vi "Test Filter Parametrized Test Cases.vi"(11 "Test Case In":refnum<class "Parameterized Test Case Test.lvclass">) -> (0 "error out":errorcluster, 3 "Test Case Out":refnum<class "Parameterized Test Case Test.lvclass">)   [LabVIEW 2020, in "Parameterized Test Case Test.lvclass"]
uses:
  Parameterized Test Case Test.lvclass
  C:/Program Files (x86)/National Instruments/LabVIEW 2020/vi.lib/Astemes/LUnit/Test Case.lvclass
  <vilib>/Astemes/LUnit/Test Case.lvclass/Test Case.ctl
  399136ac-e113-4bca-be3a-8dde4e32c814.vi
  <vilib>/Astemes/LUnit/Palette/Pass If.vi
  <vilib>/Astemes/LUnit/Append Fail Result.vi
  <vilib>/Astemes/LUnit/Append Pass Result.vi
  <vilib>/Astemes/LUnit/Run In UI.vi
  <vilib>/Utility/error.llb/Clear Errors.vi
  source/Parameterized Test Case/Parameterized Test Case.lvclass
  <vilib>/Astemes/LUnit/Test Suite.lvclass
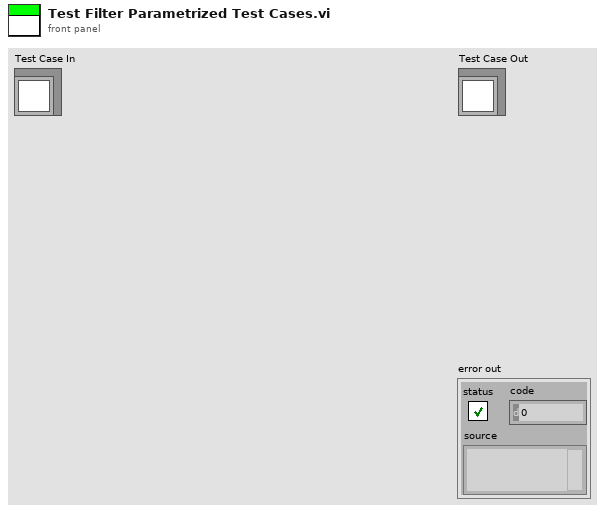
[diagram p1: front panel]
types:
  T1 = cluster{"Name":string, "Message":string, "Description":string, "Status":enum16{"", "Passed", "Failed", "Error", "Skipped", "Setup Error", "Broken", "Teardown Error"}, "Result Type":enum16{"Test Case", "Test Suite", "Test Run", "Pass", "Fail", "Skip", "Pass if", "Fail if", "Pass if Error", "Fail if Error", "Pass if Equal", "Fail if Equal"}, "Execution Time":dbl}[]
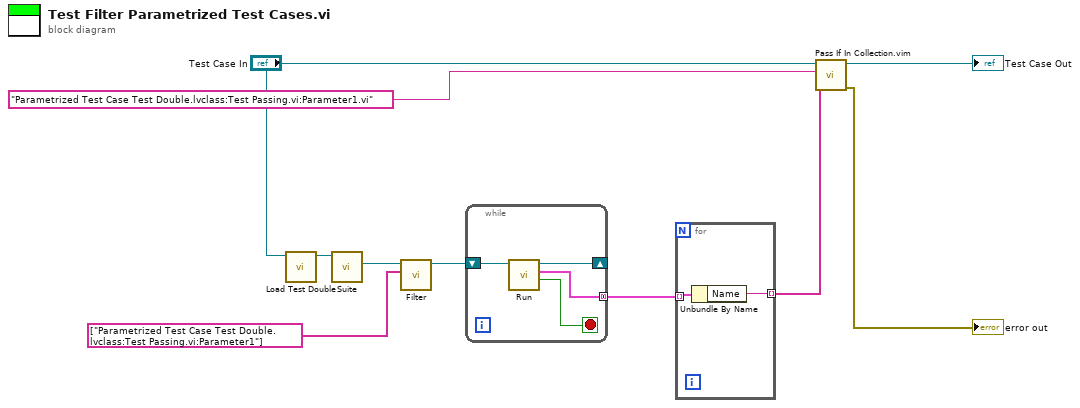
[diagram p0: block diagram]
diagram:
  n1 = call "Load Test Double.vi"("Parameterized Test Case Test in"="Test Case In") -> ("Parameterized Test Case out"=w1:refnum<class "Parameterized Test Case.lvclass">)  [unwired: 9 in, 1 out]
  n2 = call-dynamic "Suite.vi"("Parameterized Test Case In"=w1) -> ("LUnit Test Suite Out"=w7:refnum<class "Test Suite.lvclass">)  [unwired: 8 in, 2 out]
  n3 = call <vilib>:"Filter.vi"("Selected Runnables"=string[] ["Parametrized Test Case Test Double.lvclass:Test Passing.vi:Parameter1"], "LUnit Test Suite In"=w7) -> ("LUnit Test Suite Out"=w6:refnum<class "Test Suite.lvclass">)  [unwired: 8 in, 1 out]
  n4 = while {
    tunnel: [w14] -> w4 mode=concatenating
    shift-right: [w12] -> _
    shift-left: w6 -> [w13]
    stop <- w11 stop-if-true
    n5 = call-dynamic "Run.vi"("LUnit Test Suite In"=w13) -> ("Done?"=w11:bool, "Results"=w14:T1, "LUnit Test Suite In 2"=w12:refnum<class "Test Suite.lvclass">)  [unwired: 7 in, 1 out]
  }
  n6 = for {
    tunnel: w4 -> [w16] mode=indexing
    tunnel: [w15] -> w3 mode=indexing
    n7 = Unbundle By Name(w16) -> ("Name"=w15:string)
  }
  n8 = call "Pass If In Collection.vim"("Collection"=w3, "Expected Element"="Parametrized Test Case Test Double.lvclass:Test Passing.vi:Parameter1.vi" ("String"), "LUnit Test Case In"="Test Case In") -> ("error out"=→"error out":errorcluster, "LUnit Test Case Out"=→"Test Case Out":refnum<class "Parameterized Test Case Test.lvclass">)  [unwired: 7 in]
